vi "mainPage.vi"() -> ()   [LabVIEW 2018]
doc: "Use this template to build a producer/consumer design pattern with events to produce queue items. Use this design pattern instead of the User Interface Event Handler pattern for user interfaces when you want to execute code asynchronously in response to an event without slowing the user interface responsiveness."
uses:
  TypeDefs/dictCluster.ctl
  C:/Program Files (x86)/National Instruments/LabVIEW 2018/examples/Instrument IO/Serial/support/Serial - Settings.ctl
  <vilib>/Instr/_visa.llb/VISA Configure Serial Port (Instr).vi
  <vilib>/ErrorRing/Error Ring.xnode
panel:
  out "RecCmdLED":bool caption="Receiving"
  in  "service name":string="localhost"
  in  "port":u16=6969
  out "TCP FPGA Resp":string
  out "TCP Written len":i32
  in  "Send Command TCPIP":bool
  out "FPGA Resp":string
  out "UART written count":u32
  in  "Serial Settings":T1={"baud rate"=9600, "data bits"=8, "parity"=enum."None", "stop bits"=10, "flow control"=0, "VISA resource name"=""} {"flow control" items=["None"=0, "XON/XOFF"=1, "RTS/CTS"=2, "DTR/DSR"=4]; "stop bits" items=["1.0"=10, "1.5"=15, "2.0"=20]; "data bits" min=5 max=8 step=1; "baud rate" items=["75"=75, "110"=110, "134"=134, "150"=150, "300"=300, "600"=600, "1200"=1200, "1800"=1800, "2400"=2400, "4800"=4800, "7200"=7200, "9600"=9600, "14400"=14400, "19200"=19200, "28800"=28800, "38400"=38400, "56000"=56000, "57600"=57600, "115200"=115200, "128000"=128000, "230400"=230400]}
  out "SendCmdLED":bool caption="Sending"
  out "H2F Frame":string
  in  "Sensor Array":bool[](array[boolean])
  in  "On/Off Data":bool
  out "Read Data":string
  in  "Write Data (HEX)":string
  out "Dictionary":T2
  in  "Select Macro Function":T3(radio)
  in  "Choose Command Type":T4(radio)
  in  "Additional Commands":string(combo)="40"
  in  "Channel Command":string(combo)="30"
  in  "Config & Control Command":string(combo)="20"
  in  "Information Command":string(combo)="10"
  in  "Send Command UART":bool
  in  "stop":bool
  # "DEBUGGING STUFF (Hide! Dont delete)"
  # "TCP/IP Settings"
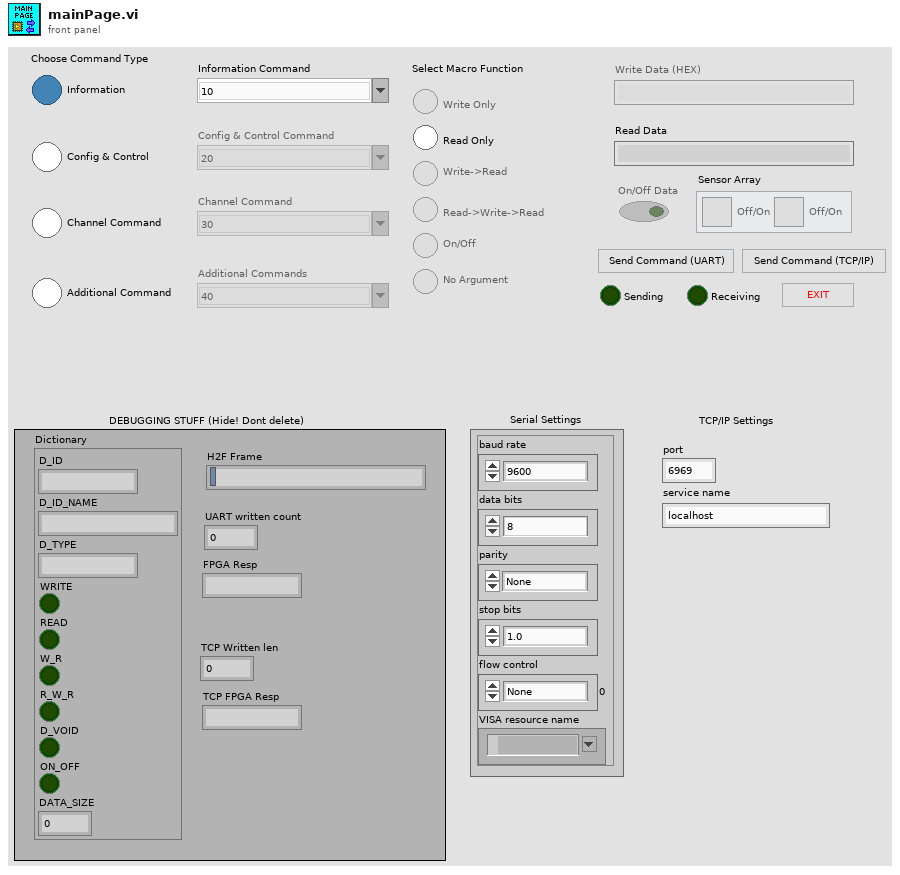
[diagram p1: front panel]
types:
  T1 = typedef "Serial - Settings.ctl" = cluster{"baud rate":u32, "data bits":u16, "parity":enum16{"None", "Odd", "Even", "Mark", "Space"}, "stop bits":u16, "flow control":u16, "VISA resource name":refnum<visa-resource-name>}
  T2 = typedef "dictCluster.ctl" = cluster{"D_ID":string, "D_ID_NAME":string, "D_TYPE":string, "WRITE":bool, "READ":bool, "W_R":bool, "R_W_R":bool, "D_VOID":bool, "ON_OFF":bool, "DATA_SIZE":u8}
  T3 = enum32{"No Selection", "WRITE", "READ", "WRITE -> READ", "READ -> WRITE -> READ", "ON/OFF", "NO ARGS"}
  T4 = enum32{"Information", "Config&Control", "Channel", "Additional"}
  T5 = enum8{"Enabled", "Disabled", "Disabled and Grayed Out"}
  T6 = cluster{"D_ID":string, "D_ID_NAME":string, "D_TYPE":string, "WRITE":bool, "READ":bool, "W_R":bool, "R_W_R":bool, "D_VOID":bool, "ON_OFF":bool, "DATA_SIZE":u8}
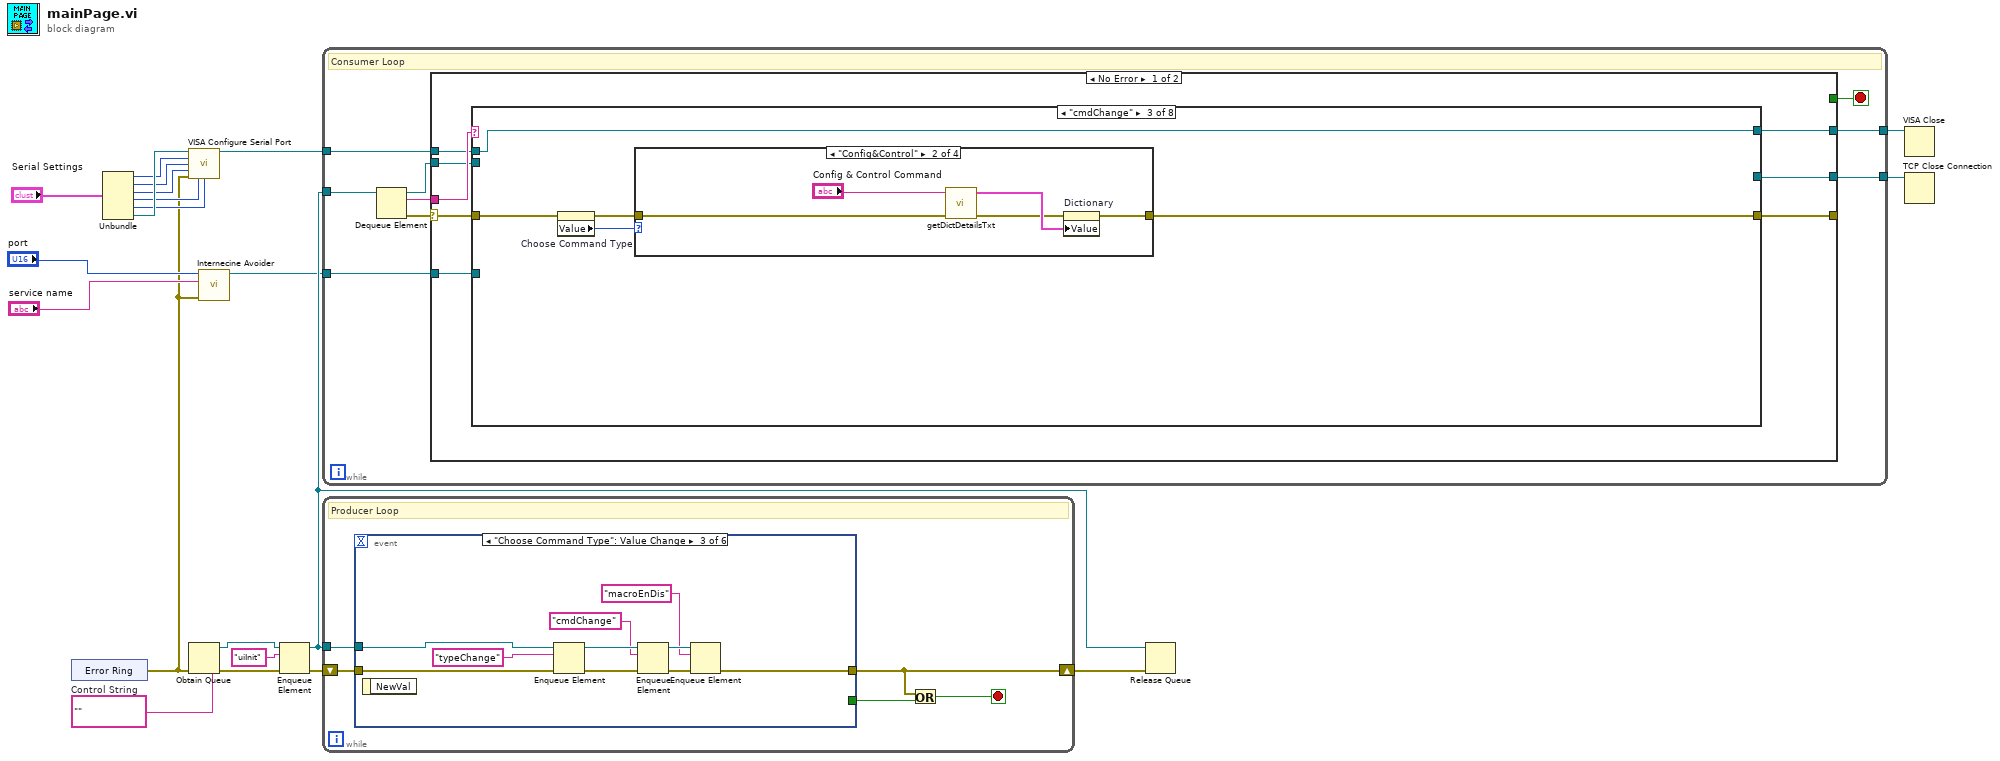
[diagram p0: block diagram]
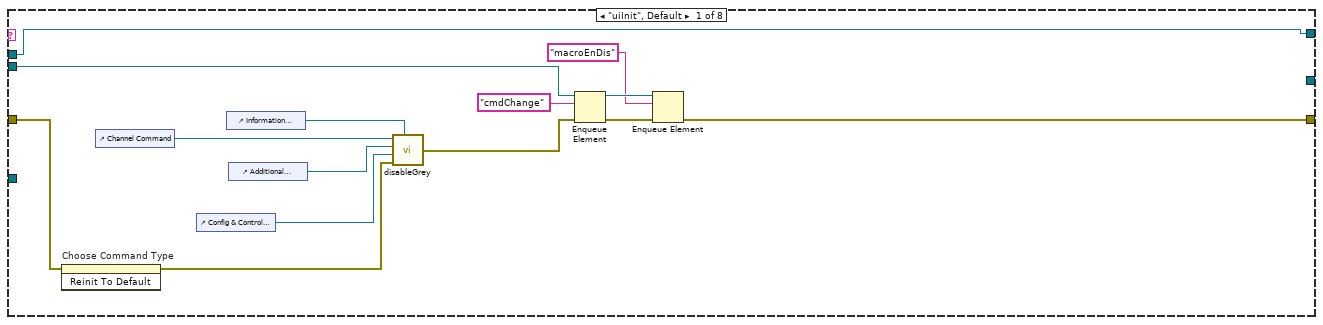
[diagram p2: hidden frame]
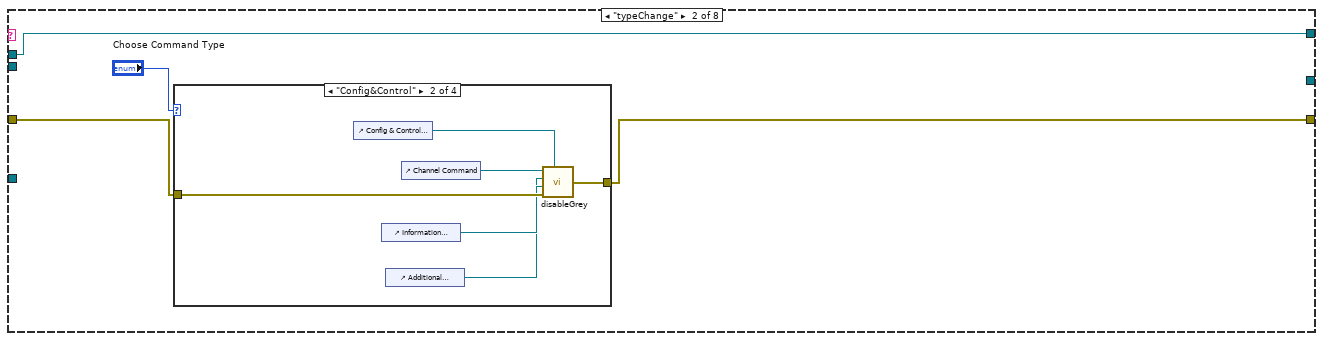
[diagram p3: hidden frame]
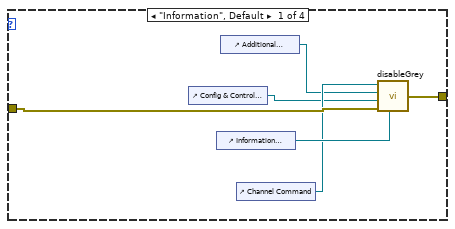
[diagram p4: hidden frame]
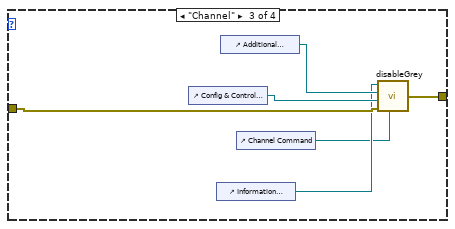
[diagram p5: hidden frame]
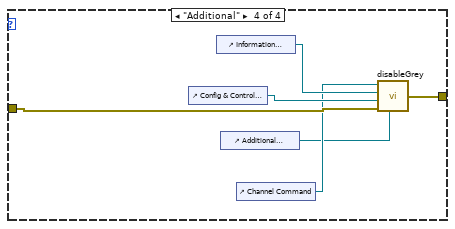
[diagram p6: hidden frame]
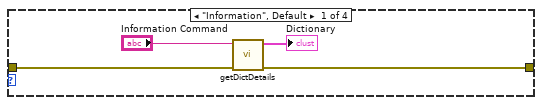
[diagram p7: hidden frame]
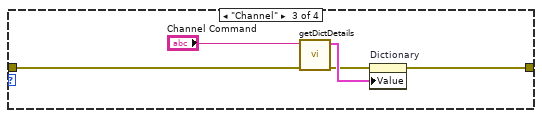
[diagram p8: hidden frame]
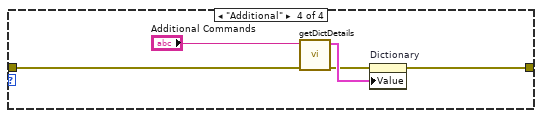
[diagram p9: hidden frame]
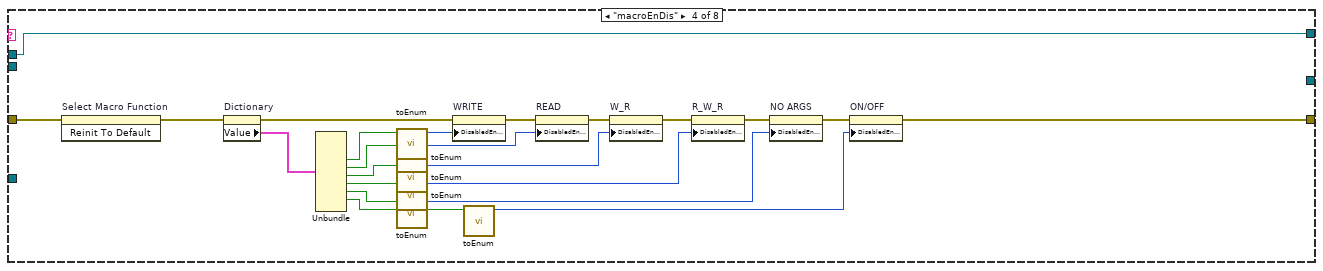
[diagram p10: hidden frame]
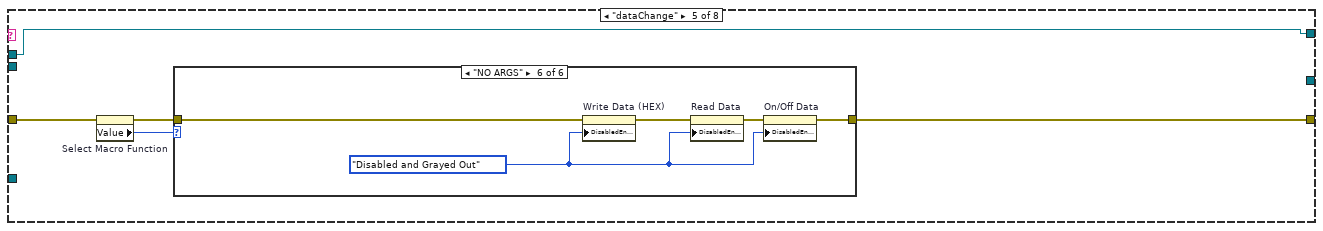
[diagram p11: hidden frame]
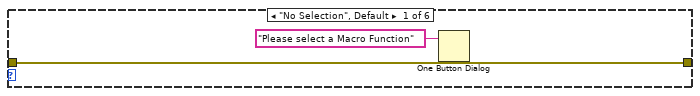
[diagram p12: hidden frame]
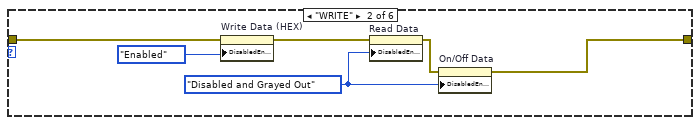
[diagram p13: hidden frame]
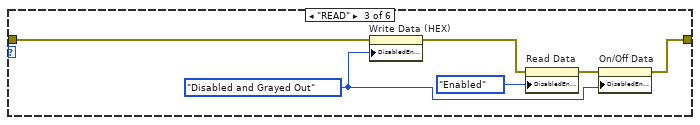
[diagram p14: hidden frame]
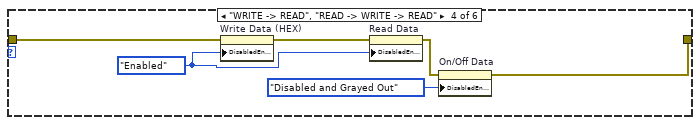
[diagram p15: hidden frame]
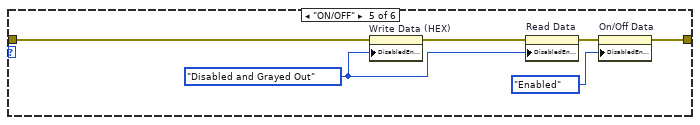
[diagram p16: hidden frame]
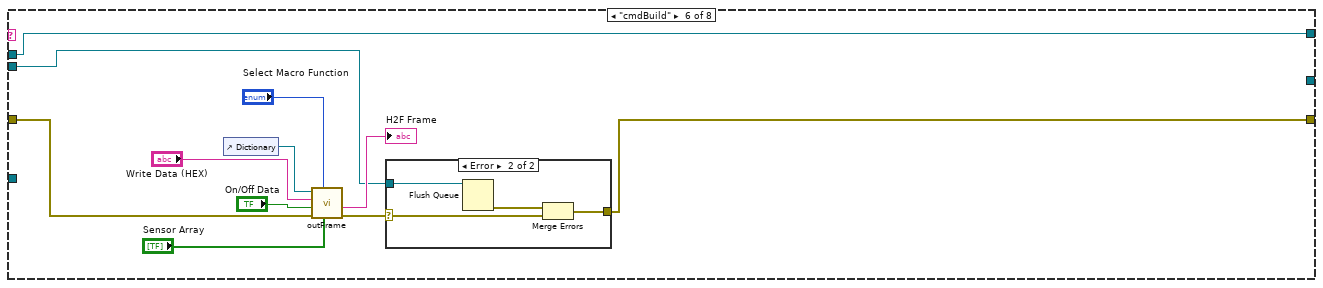
[diagram p17: hidden frame]
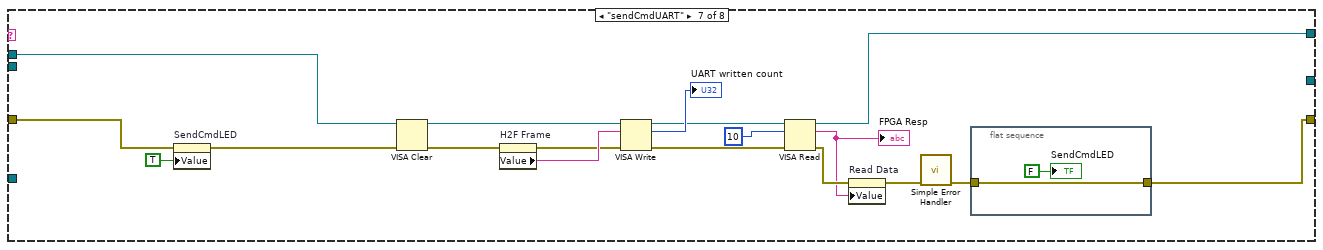
[diagram p19: hidden frame]
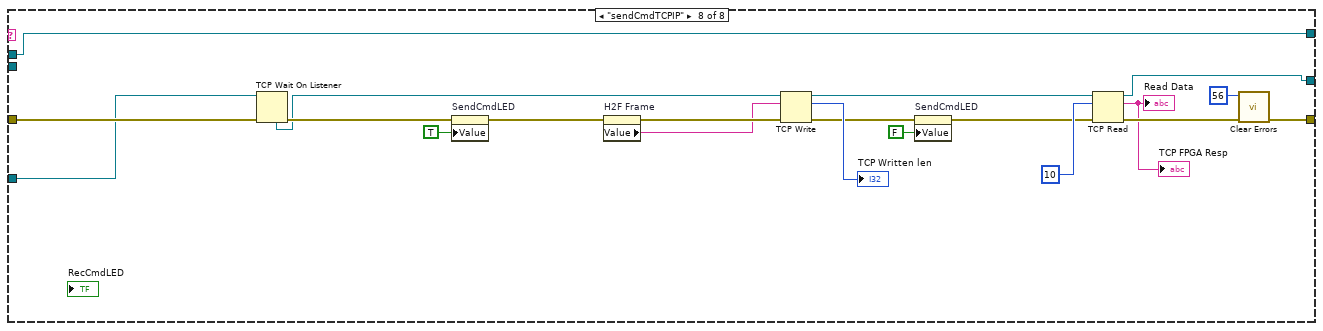
[diagram p20: hidden frame]
diagram:
  w11 = ""  # Control String
  n1 = xnode "Error Ring"() -> ("error out"=w2:errorcluster)
  n2 = Unbundle("Serial Settings") -> ("baud rate"=w15:u32, "data bits"=w16:u16, "parity"=w17:enum16{"None", "Odd", "Even", "Mark", "Space"}, "stop bits"=w18:u16, "flow control"=w12:u16, "VISA resource name"=w19:refnum<visa-resource-name>)
  n3 = call-poly "VISA Configure Serial Port"("VISA resource name"=w19, "baud rate (9600)"=w15, "data bits (8)"=w16, "parity (0:none)"=w17, "error in (no error)"=w2, "stop bits (10: 1 bit)"=w18, "flow control (0:none)"=w12) -> ("VISA resource name out"=w13:refnum<visa-resource-name>)  [unwired: 7 in, 1 out]
  n4 = Obtain Queue(element data type=w11, error in (no error)=w2) -> (queue out=w20:refnum<queue>, error out=w9:errorcluster)  [unwired: 3 in, 1 out]
  n5 = call <vilib>:"Internecine Avoider.vi"("error in"=w2, "service name"="service name", "port"="port") -> ("connection ID"=w1:refnum<k5>)  [unwired: 1 in, 7 out]
  n6 = Enqueue Element(queue=w20, element="uiInit", error in (no error)=w9) -> (queue out=w10:refnum<queue>, error out=w8:errorcluster)  [unwired: 1 in, 1 out]
  n7 = while {
    tunnel: w10 -> [w30]
    tunnel: w13 -> [w26]
    tunnel: [w24] -> w6
    tunnel: [w23] -> w5
    tunnel: w1 -> [w22]
    stop <- w27 stop-if-true
    # "Consumer Loop"
    n8 = Dequeue Element(queue=w30) -> (queue out=w25:refnum<queue>, element=w28:string, error out=w29:errorcluster)  [unwired: 2 in, 1 out]
    n9 = case shown="No Error" w29 {
      selector: w29 -> [w35 w222]
      tunnel: w28 -> [w38 _]
      tunnel: [w37 w222] -> _
      tunnel: [_ TRUE] -> w27
      tunnel: w26 -> [w36 w220]
      tunnel: w25 -> [w34 _]
      tunnel: [w33 _] -> w24
      tunnel: [w32 w220] -> w23
      tunnel: w22 -> [w31 _]
      frame No Error {
        n10 = case shown="\"cmdChange\"" w38 {
          tunnel: w35 -> [w52 w55 w85 w108 w132 w174 w197 w203]
          tunnel: [w42 w54 w82 w109 w130 w165 w188 w208] -> w37
          tunnel: w36 -> [w39 w53 w81 w105 w128 w164 w190 w205]
          tunnel: w34 -> [w44 _ _ _ _ w166 _ _]
          tunnel: [_ _ _ _ _ _ _ w206] -> w33
          tunnel: [w39 w53 w81 w105 w128 w164 w183 w205] -> w32
          tunnel: w31 -> [_ _ _ _ _ _ _ w201]
          frame "uiInit", Default {
            n11 = invoke on="Choose Command Type" class="RadioBtnsControl (strict)" method="Reinit To Default"(error in=w52) -> (error out=w47:errorcluster)  [unwired: 2 in, 2 out]
            n12 = control-ref of="Channel Command"() -> (w50:refnum<vi>)
            n13 = control-ref of="Config & Control Command"() -> (w48:refnum<vi>)
            n14 = control-ref of="Information Command"() -> (w51:refnum<vi>)
            n15 = control-ref of="Additional Commands"() -> (w49:refnum<vi>)
            n16 = call "disableGrey.vi"("Disable 1"=w50, "Disable 2"=w49, "Disable 3"=w48, "error in (no error)"=w47, "Enable this"=w51) -> ("error out"=w46:errorcluster)
            n17 = Enqueue Element(queue=w44, element="cmdChange", error in (no error)=w46) -> (queue out=w41:refnum<queue>, error out=w45:errorcluster)  [unwired: 1 in, 1 out]
            n18 = Enqueue Element(queue=w41, element="macroEnDis", error in (no error)=w45) -> (error out=w42:errorcluster)  [unwired: 1 in, 2 out]
          }
          frame "typeChange" {
            n19 = case shown="\"Config&Control\"" "Choose Command Type" {
              tunnel: w55 -> [w62 w68 w74 w79]
              tunnel: [w57 w67 w73 w80] -> w54
              frame "Information", Default {
                n20 = control-ref of="Config & Control Command"() -> (w58:refnum<vi>)
                n21 = control-ref of="Information Command"() -> (w61:refnum<vi>)
                n22 = control-ref of="Additional Commands"() -> (w59:refnum<vi>)
                n23 = control-ref of="Channel Command"() -> (w60:refnum<vi>)
                n24 = call "disableGrey.vi"("Disable 1"=w60, "Disable 2"=w59, "Disable 3"=w58, "error in (no error)"=w62, "Enable this"=w61) -> ("error out"=w57:errorcluster)
              }
              frame "Config&Control" {
                n25 = control-ref of="Config & Control Command"() -> (w63:refnum<vi>)
                n26 = control-ref of="Information Command"() -> (w66:refnum<vi>)
                n27 = control-ref of="Additional Commands"() -> (w65:refnum<vi>)
                n28 = control-ref of="Channel Command"() -> (w64:refnum<vi>)
                n29 = call "disableGrey.vi"("Disable 1"=w64, "Disable 2"=w65, "Disable 3"=w66, "error in (no error)"=w68, "Enable this"=w63) -> ("error out"=w67:errorcluster)
              }
              frame "Channel" {
                n30 = control-ref of="Config & Control Command"() -> (w72:refnum<vi>)
                n31 = control-ref of="Information Command"() -> (w70:refnum<vi>)
                n32 = control-ref of="Additional Commands"() -> (w71:refnum<vi>)
                n33 = control-ref of="Channel Command"() -> (w69:refnum<vi>)
                n34 = call "disableGrey.vi"("Disable 1"=w70, "Disable 2"=w71, "Disable 3"=w72, "error in (no error)"=w74, "Enable this"=w69) -> ("error out"=w73:errorcluster)
              }
              frame "Additional" {
                n35 = control-ref of="Config & Control Command"() -> (w78:refnum<vi>)
                n36 = control-ref of="Information Command"() -> (w77:refnum<vi>)
                n37 = control-ref of="Additional Commands"() -> (w75:refnum<vi>)
                n38 = control-ref of="Channel Command"() -> (w76:refnum<vi>)
                n39 = call "disableGrey.vi"("Disable 1"=w76, "Disable 2"=w77, "Disable 3"=w78, "error in (no error)"=w79, "Enable this"=w75) -> ("error out"=w80:errorcluster)
              }
            }
          }
          frame "cmdChange" {
            n40 = property on="Choose Command Type" class="RadioBtnsControl (strict)"(error in=w85) -> (error out=w83:errorcluster, "Value"=w84:T4)  [unwired: 1 in, 1 out]
            n41 = case shown="\"Config&Control\"" w84 {
              tunnel: w83 -> [w88 w92 w99 w104]
              tunnel: [w86 w94 w95 w100] -> w82
              frame "Information", Default {
                n42 = call "getDictDetails.vi"("error in (no error)"=w88, "Dictionary ID Input"="Information Command") -> ("error out"=w86:errorcluster, "Dictionary"=→"Dictionary":T6)  [unwired: 8 in]
              }
              frame "Config&Control" {
                n43 = call "getDictDetailsTxt.vi"("error constant"=w92, "Dictionary ID Input"="Config & Control Command") -> ("error IO"=w90:errorcluster, "Dictionary"=w91:T6)  [unwired: 8 in]
                n44 = property on="Dictionary" class="Clust (strict)"(error in=w90, "Value"=w91) -> (error out=w94:errorcluster)  [unwired: 1 in, 1 out]
              }
              frame "Channel" {
                n45 = call "getDictDetails.vi"("error in (no error)"=w99, "Dictionary ID Input"="Channel Command") -> ("error out"=w96:errorcluster, "Dictionary"=w97:T6)  [unwired: 8 in]
                n46 = property on="Dictionary" class="Clust (strict)"(error in=w96, "Value"=w97) -> (error out=w95:errorcluster)  [unwired: 1 in, 1 out]
              }
              frame "Additional" {
                n47 = call "getDictDetails.vi"("error in (no error)"=w104, "Dictionary ID Input"="Additional Commands") -> ("error out"=w101:errorcluster, "Dictionary"=w102:T6)  [unwired: 8 in]
                n48 = property on="Dictionary" class="Clust (strict)"(error in=w101, "Value"=w102) -> (error out=w100:errorcluster)  [unwired: 1 in, 1 out]
              }
            }
          }
          frame "macroEnDis" {
            n49 = invoke on="Select Macro Function" class="RadioBtnsControl (strict)" method="Reinit To Default"(error in=w108) -> (error out=w107:errorcluster)  [unwired: 2 in, 2 out]
            n50 = property on="Dictionary" class="Clust (strict)"(error in=w107) -> (error out=w115:errorcluster, "Value"=w127:T2)  [unwired: 1 in, 1 out]
            n51 = Unbundle(w127) -> ("WRITE"=w126:bool, "READ"=w125:bool, "W_R"=w124:bool, "R_W_R"=w123:bool, "D_VOID"=w122:bool, "ON_OFF"=w121:bool)  [unwired: 4 out]
            n52 = call "toEnum.vi"("Instruction"=w126) -> ("Enable/Disable?"=w106:u8)  [unwired: 10 in]
            n53 = call "toEnum.vi"("Instruction"=w125) -> ("Enable/Disable?"=w116:u8)  [unwired: 10 in]
            n54 = call "toEnum.vi"("Instruction"=w124) -> ("Enable/Disable?"=w117:u8)  [unwired: 10 in]
            n55 = call "toEnum.vi"("Instruction"=w123) -> ("Enable/Disable?"=w118:u8)  [unwired: 10 in]
            n56 = call "toEnum.vi"("Instruction"=w122) -> ("Enable/Disable?"=w119:u8)  [unwired: 10 in]
            n57 = property on="WRITE" class="Bool (strict)"(error in=w115, "DisabledEnum"=w106) -> (error out=w114:errorcluster)  [unwired: 1 in, 1 out]
            n58 = call "toEnum.vi"("Instruction"=w121) -> ("Enable/Disable?"=w120:u8)  [unwired: 10 in]
            n59 = property on="READ" class="Bool (strict)"(error in=w114, "DisabledEnum"=w116) -> (error out=w113:errorcluster)  [unwired: 1 in, 1 out]
            n60 = property on="W_R" class="Bool (strict)"(error in=w113, "DisabledEnum"=w117) -> (error out=w112:errorcluster)  [unwired: 1 in, 1 out]
            n61 = property on="R_W_R" class="Bool (strict)"(error in=w112, "DisabledEnum"=w118) -> (error out=w111:errorcluster)  [unwired: 1 in, 1 out]
            n62 = property on="NO ARGS" class="Bool (strict)"(error in=w111, "DisabledEnum"=w119) -> (error out=w110:errorcluster)  [unwired: 1 in, 1 out]
            n63 = property on="ON/OFF" class="Bool (strict)"(error in=w110, "DisabledEnum"=w120) -> (error out=w109:errorcluster)  [unwired: 1 in, 1 out]
          }
          frame "dataChange" {
            n64 = property on="Select Macro Function" class="RadioBtnsControl (strict)"(error in=w132) -> (error out=w129:errorcluster, "Value"=w131:T3)  [unwired: 1 in, 1 out]
            n65 = case shown="\"NO ARGS\"" w131 {
              tunnel: w129 -> [w133 w138 w142 w148 w154 w160]
              tunnel: [w133 w137 w141 w147 w153 w159] -> w130
              frame "No Selection", Default {
                n66 = One Button Dialog(message="Please select a Macro Function") -> ()  [unwired: 1 in, 1 out]
              }
              frame "WRITE" {
                w135 = T5."Disabled and Grayed Out" ("Disabled")
                n67 = property on="Write Data (HEX)" class="Str"(error in=w138, "DisabledEnum"=T5."Enabled" ("Disabled")) -> (error out=w140:errorcluster)  [unwired: 1 in, 1 out]
                n68 = property on="Read Data" class="Str"(error in=w140, "DisabledEnum"=w135) -> (error out=w139:errorcluster)  [unwired: 1 in, 1 out]
                n69 = property on="On/Off Data" class="Bool (strict)"(error in=w139, "DisabledEnum"=w135) -> (error out=w137:errorcluster)  [unwired: 1 in, 1 out]
              }
              frame "READ" {
                w143 = T5."Disabled and Grayed Out" ("Disabled")
                n70 = property on="Write Data (HEX)" class="Str"(error in=w142, "DisabledEnum"=w143) -> (error out=w146:errorcluster)  [unwired: 1 in, 1 out]
                n71 = property on="Read Data" class="Str"(error in=w146, "DisabledEnum"=T5."Enabled" ("Disabled")) -> (error out=w145:errorcluster)  [unwired: 1 in, 1 out]
                n72 = property on="On/Off Data" class="Bool (strict)"(error in=w145, "DisabledEnum"=w143) -> (error out=w141:errorcluster)  [unwired: 1 in, 1 out]
              }
              frame "WRITE -> READ", "READ -> WRITE -> READ" {
                w149 = T5."Enabled" ("Disabled")
                n73 = property on="Write Data (HEX)" class="Str"(error in=w148, "DisabledEnum"=w149) -> (error out=w152:errorcluster)  [unwired: 1 in, 1 out]
                n74 = property on="Read Data" class="Str"(error in=w152, "DisabledEnum"=w149) -> (error out=w151:errorcluster)  [unwired: 1 in, 1 out]
                n75 = property on="On/Off Data" class="Bool (strict)"(error in=w151, "DisabledEnum"=T5."Disabled and Grayed Out" ("Disabled")) -> (error out=w147:errorcluster)  [unwired: 1 in, 1 out]
              }
              frame "ON/OFF" {
                w156 = T5."Disabled and Grayed Out" ("Disabled")
                n76 = property on="Write Data (HEX)" class="Str"(error in=w154, "DisabledEnum"=w156) -> (error out=w158:errorcluster)  [unwired: 1 in, 1 out]
                n77 = property on="Read Data" class="Str"(error in=w158, "DisabledEnum"=w156) -> (error out=w157:errorcluster)  [unwired: 1 in, 1 out]
                n78 = property on="On/Off Data" class="Bool (strict)"(error in=w157, "DisabledEnum"=T5."Enabled" ("Disabled")) -> (error out=w153:errorcluster)  [unwired: 1 in, 1 out]
              }
              frame "NO ARGS" {
                w161 = T5."Disabled and Grayed Out" ("Disabled")
                n79 = property on="Write Data (HEX)" class="Str"(error in=w160, "DisabledEnum"=w161) -> (error out=w163:errorcluster)  [unwired: 1 in, 1 out]
                n80 = property on="Read Data" class="Str"(error in=w163, "DisabledEnum"=w161) -> (error out=w162:errorcluster)  [unwired: 1 in, 1 out]
                n81 = property on="On/Off Data" class="Bool (strict)"(error in=w162, "DisabledEnum"=w161) -> (error out=w159:errorcluster)  [unwired: 1 in, 1 out]
              }
            }
          }
          frame "cmdBuild" {
            n82 = control-ref of="Dictionary"() -> (w170:refnum<vi>)
            n83 = call "outFrame.vi"("Sensor Array"="Sensor Array", "Select Macro Function"="Select Macro Function", "error in (no error)"=w174, "On/Off Data"="On/Off Data", "Write Data (HEX)"="Write Data (HEX)", "Cluster in"=w170) -> ("error out"=w167:errorcluster, "H2F Frame"=→"H2F Frame":string)  [unwired: 4 in]
            n84 = case shown="Error" w167 {
              selector: w167 -> [w175 w176]
              tunnel: [w175 w178] -> w165
              tunnel: w166 -> [_ w179]
              frame No Error {
              }
              frame Error {
                n85 = Flush Queue(queue=w179) -> (error out=w177:errorcluster)  [unwired: 1 in, 2 out]
                n86 = Merge Errors(w177, w176) -> (w178:errorcluster)
              }
            }
          }
          frame "sendCmdUART" {
            n87 = property on="SendCmdLED" class="Bool (strict)"(error in=w197, "Value"=TRUE ("Sending Command")) -> (error out=w189:errorcluster)  [unwired: 1 in, 1 out]
            n88 = VISA Clear(VISA resource name=w190, error in (no error)=w189) -> (VISA resource name out=w191:refnum<visa-resource-name>, error out=w192:errorcluster)
            n89 = property on="H2F Frame" class="Str"(error in=w192) -> (error out=w194:errorcluster, "Value"=w195:string)  [unwired: 1 in, 1 out]
            n90 = VISA Write(VISA resource name=w191, write buffer=w195, error in (no error)=w194) -> (VISA resource name out=w186:refnum<visa-resource-name>, return count=→"UART written count":u32, error out=w184:errorcluster)
            n91 = VISA Read(VISA resource name=w186, byte count=u32 10, error in (no error)=w184) -> (VISA resource name out=w183:refnum<visa-resource-name>, read buffer=w180:string, error out=w181:errorcluster)  [unwired: 1 out]
            "FPGA Resp" <- w180
            n92 = property on="Read Data" class="Str"(error in=w181, "Value"=w180) -> (error out=w182:errorcluster)  [unwired: 1 in, 1 out]
            n93 = call <vilib>:"Simple Error Handler.vi"("error in (no error)"=w182) -> ("error out"=w187:errorcluster)  [unwired: 4 in, 4 out]
            n94 = flat-sequence {
              tunnel: [w198] -> w188
              tunnel: w187 -> [w198]
              frame #0 {
                "SendCmdLED" <- FALSE ("Sending Command")
              }
            }
          }
          frame "sendCmdTCPIP" {
            n95 = TCP Wait On Listener(8:w203, 11:w201) -> (0:w202:errorcluster, 4:w200:refnum<k5>)  [unwired: 2 in, 3 out]
            n96 = property on="SendCmdLED" class="Bool (strict)"(error in=w202, "Value"=TRUE ("Sending Command")) -> (error out=w215:errorcluster)  [unwired: 1 in, 1 out]
            n97 = property on="H2F Frame" class="Str"(error in=w215) -> (error out=w219:errorcluster, "Value"=w218:string)  [unwired: 1 in, 1 out]
            n98 = TCP Write(connection ID=w200, data in=w218, error in (no error)=w219) -> (connection ID out=w214:refnum<k5>, bytes written=→"TCP Written len":i32, error out=w211:errorcluster)  [unwired: 1 in]
            n99 = property on="SendCmdLED" class="Bool (strict)"(error in=w211, "Value"=FALSE ("Sending Command")) -> (error out=w210:errorcluster)  [unwired: 1 in, 1 out]
            n100 = TCP Read(connection ID=w214, bytes to read=10, error in (no error)=w210) -> (connection ID out=w206:refnum<k5>, data out=→"TCP FPGA Resp" →"Read Data":string, error out=w209:errorcluster)  [unwired: 2 in]
            n101 = call <vilib>:"Clear Errors.vi"("error in (no error)"=w209, "specific error code to clear (0: all)"=56) -> ("error out"=w208:errorcluster)  [unwired: 4 in, 1 out]
          }
        }
      }
      frame Error {
        # "Return true in any case that should stop the loop."
      }
    }
  }
  n102 = while {
    shift-right: [w223] -> w21
    shift-left: w8 -> [w226]
    tunnel: w10 -> [w227]
    stop <- w224 stop-if-true
    # "Producer Loop"
    n103 = event shown="[2] \"Choose Command Type\": Value Change" {
      selector: _ -> [_ _ _ _ _ _]
      dyn-events: _ -> [_ _ _ _ _ _]
      timeout: _ -> [_ _ _ _ _ _]
      tunnel: w227 -> [w234 w241 w250 w258 _ w262]
      tunnel: w226 -> [w232 w239 w249 w257 w259 w264]
      tunnel: [w230 w237 w244 w255 w259 w263] -> w223
      tunnel: [_ _ _ _ "stop" _] -> w225
      event "Send Command UART": Value Change {
        n104 = event-data() -> ()  [unwired: 1 in, 1 out]
        n105 = Enqueue Element(queue=w234, element="cmdBuild", error in (no error)=w232) -> (queue out=w229:refnum<queue>, error out=w233:errorcluster)  [unwired: 1 in, 1 out]
        n106 = Enqueue Element(queue=w229, element="sendCmdUART", error in (no error)=w233) -> (error out=w230:errorcluster)  [unwired: 1 in, 2 out]
      }
      event "Send Command TCPIP": Value Change {
        n107 = event-data() -> ()  [unwired: 1 in, 1 out]
        n108 = Enqueue Element(queue=w241, element="cmdBuild", error in (no error)=w239) -> (queue out=w236:refnum<queue>, error out=w240:errorcluster)  [unwired: 1 in, 1 out]
        n109 = Enqueue Element(queue=w236, element="sendCmdTCPIP", error in (no error)=w240) -> (error out=w237:errorcluster)  [unwired: 1 in, 2 out]
      }
      event "Choose Command Type": Value Change {
        n110 = event-data() -> ()  [unwired: 1 in, 1 out]
        n111 = Enqueue Element(queue=w250, element="typeChange", error in (no error)=w249) -> (queue out=w246:refnum<queue>, error out=w251:errorcluster)  [unwired: 1 in, 1 out]
        n112 = Enqueue Element(queue=w246, element="cmdChange", error in (no error)=w251) -> (queue out=w243:refnum<queue>, error out=w247:errorcluster)  [unwired: 1 in, 1 out]
        n113 = Enqueue Element(queue=w243, element="macroEnDis", error in (no error)=w247) -> (error out=w244:errorcluster)  [unwired: 1 in, 2 out]
      }
      event "Information Command", "Config & Control Command", "Additional Commands", "Channel Command": Value Change {
        n114 = event-data() -> ()  [unwired: 1 in, 1 out]
        n115 = Enqueue Element(queue=w258, element="cmdChange", error in (no error)=w257) -> (queue out=w252:refnum<queue>, error out=w254:errorcluster)  [unwired: 1 in, 1 out]
        n116 = Enqueue Element(queue=w252, element="macroEnDis", error in (no error)=w254) -> (error out=w255:errorcluster)  [unwired: 1 in, 2 out]
      }
      event "stop": Value Change {
        n117 = event-data() -> ()  [unwired: 1 in, 1 out]
      }
      event "Select Macro Function": Value Change {
        n118 = event-data() -> ()  [unwired: 1 in, 1 out]
        n119 = Enqueue Element(queue=w262, element="dataChange", error in (no error)=w264) -> (error out=w263:errorcluster)  [unwired: 1 in, 2 out]
      }
    }
    n120 = Or(x=w223, y=w225) -> (x .or. y?=w224:bool)
  }
  n121 = Release Queue(queue=w10, error in (no error)=w21) -> ()  [unwired: 1 in, 3 out]
  n122 = VISA Close(VISA resource name=w5) -> ()  [unwired: 1 in, 1 out]
  n123 = TCP Close Connection(connection ID=w6) -> ()  [unwired: 1 in, 3 out]
